vi "Set_Container.vi"(8 "error in (no error)":errorcluster, 10 "data":T1, 11 "IB_Source_Container in":refnum<class "IB_Source_Container.lvclass">) -> (0 "error out":errorcluster, 3 "IB_Source_Container out":refnum<class "IB_Source_Container.lvclass">)   [LabVIEW 2020, in "IB_Source_Container.lvclass"]
uses:
  <vilib>/AppBuilder/IB_Classes/Source/Container/IB_Source_Container.lvclass
  <vilib>/AppBuilder/IB_Classes/Source/Container/IB_Source_Container.lvclass/IB_Source_Container.ctl
  <vilib>/AppBuilder/IB_Classes/Source/Container/IB_Source_Container.ctl
  <vilib>/AppBuilder/IB_Classes/Source/File/CtrFile/IB_CtrFile.lvclass
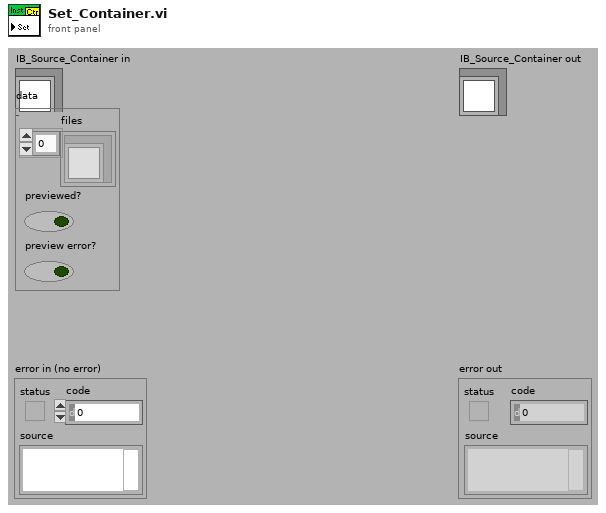
[diagram p1: front panel]
types:
  T1 = typedef "IB_Source_Container.ctl" = cluster{"files":refnum<class "IB_CtrFile.lvclass">[], "previewed?":bool, "preview error?":bool}
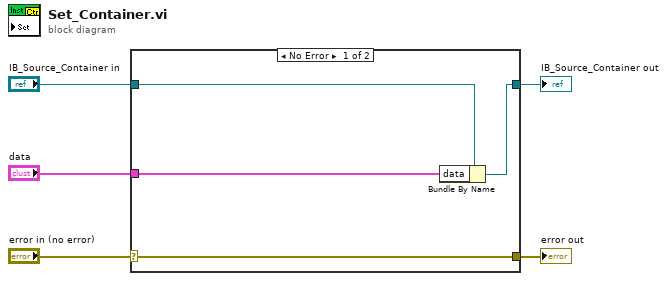
[diagram p0: block diagram]
diagram:
  n1 = case shown="No Error" "error in (no error)" {
    selector: "error in (no error)" -> [w9 w10]
    tunnel: [w9 w10] -> w4
    tunnel: [w7 w11] -> w2
    tunnel: "IB_Source_Container in" -> [w8 w11]
    tunnel: "data" -> [w6 _]
    frame No Error {
      n2 = Bundle By Name(cluster=w8, "data"=w6) -> (w7:refnum<class "IB_Source_Container.lvclass">)
    }
    frame Error {
    }
  }
  "error out" <- w4
  "IB_Source_Container out" <- w2
